vi "Stop Response Complete.vi"(8 "error in (no error)":errorcluster, 11 "Process Controller in":refnum<class "Process Controller.lvclass">) -> (0 "error out":errorcluster, 3 "Process Controller out":refnum<class "Process Controller.lvclass">)   [LabVIEW 2021, in "Process Controller.lvclass"]
uses:
  Process Controller.lvclass
  Process Controller.lvclass/Process Controller.ctl
  Publish-Subscribe/Interfaces/Publisher Messages/Unsubscribe Msg/Unsubscribe Msg.lvclass
  <vilib>/ActorFramework/Actor/Actor.lvclass
  C:/GitHub/LabActor/Worker/Worker.lvclass
  C:/GitHub/LabActor/Template Module/Template Module.lvclass
  C:/Program Files/National Instruments/LabVIEW 2021/vi.lib/ActorFramework/Actor/Actor.lvclass
  C:/GitHub/LabActor/Controllers/Process Controller/Process Controller.lvclass
  C:/GitHub/LabActor/Publish-Subscribe/Interfaces/Subscriber/Subscriber.lvclass
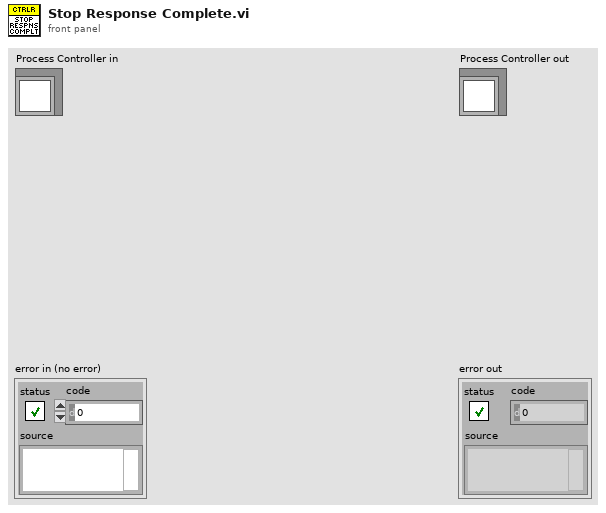
[diagram p1: front panel]
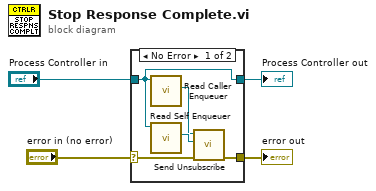
[diagram p0: block diagram]
diagram:
  n1 = case shown="No Error" "error in (no error)" {
    selector: "error in (no error)" -> [w9 w11]
    tunnel: [w8 w11] -> w3
    tunnel: [w7 w10] -> w1
    tunnel: "Process Controller in" -> [w7 w10]
    frame No Error {
      n2 = call <vilib>:"Read Caller Enqueuer.vi"("Actor"=w7) -> ("Caller Enqueuer"=w5:refnum<class "Message Enqueuer.lvclass">)  [unwired: 10 in]
      n3 = call <vilib>:"Read Self Enqueuer.vi"("Actor"=w7) -> ("Self Enqueuer"=w6:refnum<class "Message Enqueuer.lvclass">)  [unwired: 10 in]
      n4 = call "Send Unsubscribe.vi"("error in (no error)"=w9, "Subscriber Enq"=w6, "Message Enqueuer"=w5) -> ("error out"=w8:errorcluster)  [unwired: 7 in, 1 out]
    }
    frame Error {
    }
  }
  "error out" <- w3
  "Process Controller out" <- w1
